vi "Scale 4-20 sig.vi"(0 "4 mA value":dbl, 5 "20 mA value":dbl, 7 "Drop resistor":dbl) -> (4 "M":dbl, 6 "B":dbl)   [LabVIEW 2012]
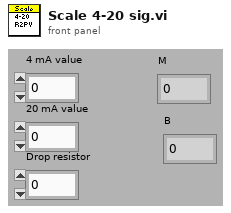
[diagram p1: front panel]
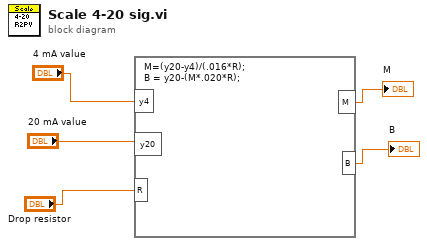
[diagram p0: block diagram]
diagram:
  n1 = formula code="M=(y20-y4)/(.016*R);\nB = y20-(M*.020*R);"("y4"="4 mA value", "y20"="20 mA value", "R"="Drop resistor") -> ("M"=→"M":dbl, "B"=→"B":dbl)
